vi "ElementToKVP.vi"(8 "error in (no error)":errorcluster, 10 "Element":variant) -> (0 "error out":errorcluster, 2 "KVP":T1)   [LabVIEW 2018, in "TestMonitor.lvclass"]
doc: "This helper VI will take in a String and return a key-value-pair for uploading to Systemlink. The key will be the name of the control, cluster element, or property you wire in, the value will be the string."
uses:
  TestMonitor.lvclass
  <vilib>/Skyline/Utilities/Property.ctl
  <vilib>/Skyline/Utilities/NI Skyline Utilities.lvlib
  <vilib>/Utility/Data Type/NI_Data Type.lvlib
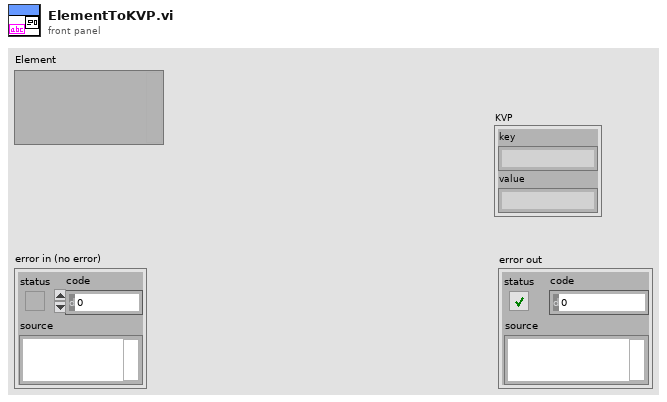
[diagram p1: front panel]
types:
  T1 = typedef "NI Skyline Utilities.lvlib/Property.ctl" = cluster{"key":string, "value":string}
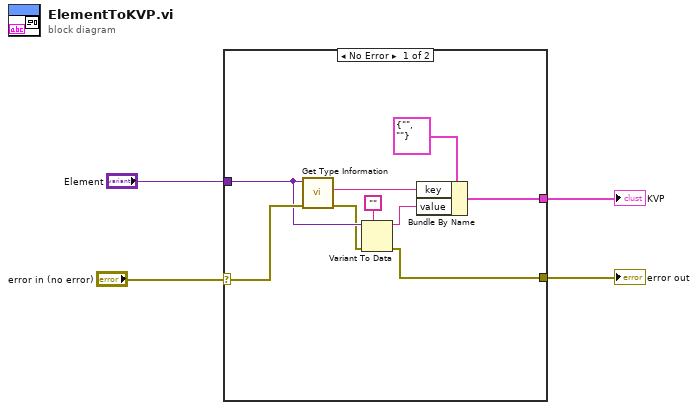
[diagram p0: block diagram]
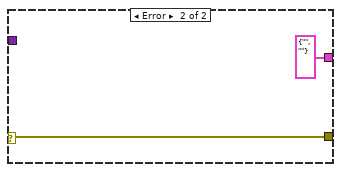
[diagram p2: hidden frame]
diagram:
  n1 = case shown="No Error" "error in (no error)" {
    selector: "error in (no error)" -> [w13 w14]
    tunnel: "Element" -> [w7 _]
    tunnel: [w10 T1 {"key"="", "value"=""} ("property")] -> w2
    tunnel: [w9 w14] -> w1
    frame No Error {
      n2 = call <vilib>:"Get Type Information.vi"("error in (no error)"=w13, "Variant"=w7) -> ("error out"=w6:errorcluster, "Name"=w11:string)  [unwired: 5 in, 3 out]
      n3 = Variant To Data(error in=w6, type="", Variant=w7) -> (data=w5:string, error out=w9:errorcluster)
      n4 = Bundle By Name(cluster=T1 {"key"="", "value"=""} ("property"), "key"=w11, "value"=w5) -> (w10:T1)
    }
    frame Error {
    }
  }
  "KVP" <- w2
  "error out" <- w1
